vi "DeviceStartupInitialisationRoutines.vi"(5 "error out 2":errorcluster) -> ()   [LabVIEW 2011]
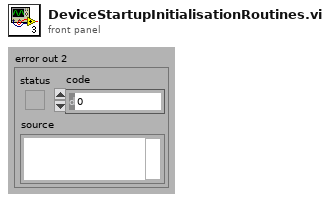
[diagram p1: front panel]
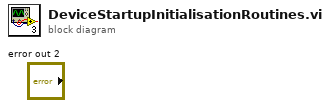
[diagram p0: block diagram]
diagram:
